vi "EF_EOG_Removal_PCA.vi"(8 "EOG":waveform(dbl)[](array[waveform]), 11 "EEG":waveform(dbl)[](array[waveform])) -> (3 "EEG out":waveform(dbl)[](array[waveform]))   [LabVIEW 2016, in "Feature Extraction.lvlib"]
uses:
  <vilib>/Analysis/baseanly.llb/Real A x B.vi
  <vilib>/addons/Time Series Analysis/Statistical Analysis.llb/TSA Principal Component Analysis (Waveform).vi
  Feature Extraction.lvlib
  <vilib>/Analysis/NI_AALBase.lvlib
  <vilib>/addons/_Advanced Signal Processing/NI_AdvSigProcTSA.lvlib
  4. Accuracy Assessment for EEG Classification/Classifier.lvlib
panel:
  out "Removed Principal Components":waveform(dbl)[](graph)
  out "Reconstructed EEG Signals":waveform(dbl)[](graph)
  out "Principal Components (PC)":waveform(dbl)[](graph)
  # "This VI is a part of BCI Design library, http://www.ru-bci.org \nCopyright © 2020, Sotnikov Peter, All rights reserved. License: GNU GPLv3"
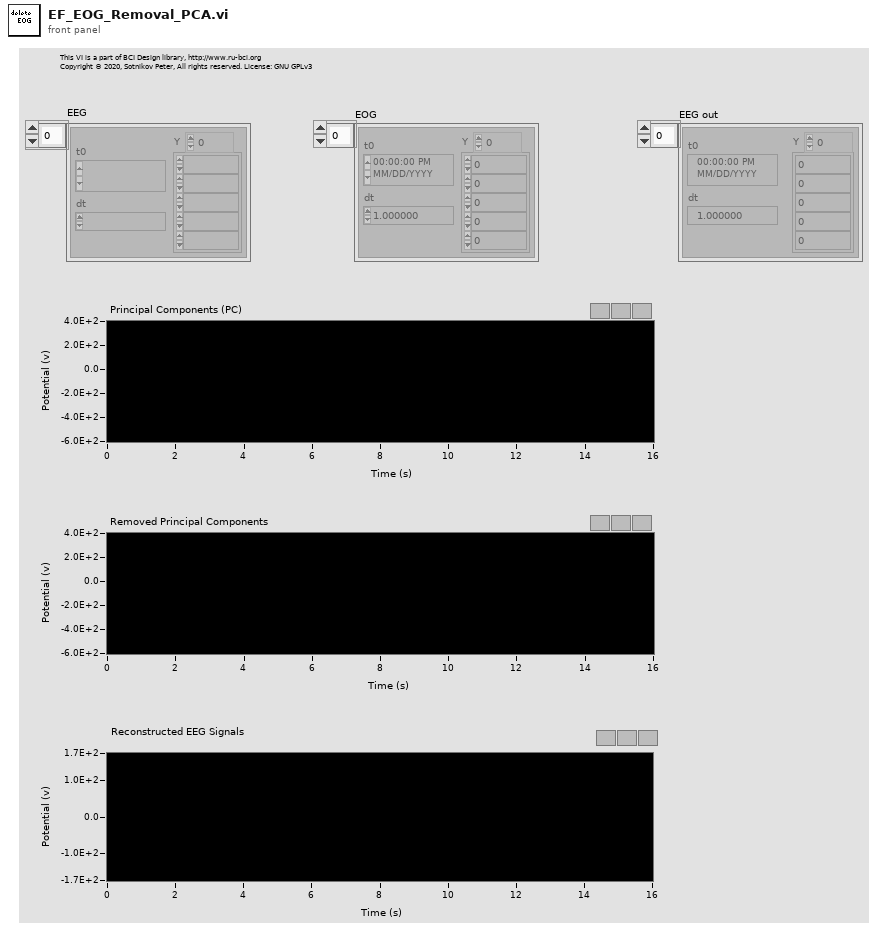
[diagram p1: front panel]
types:
  T1 = typedef "NI_Matrix.lvlib/RealMatrix.ctl" = dbl[][]
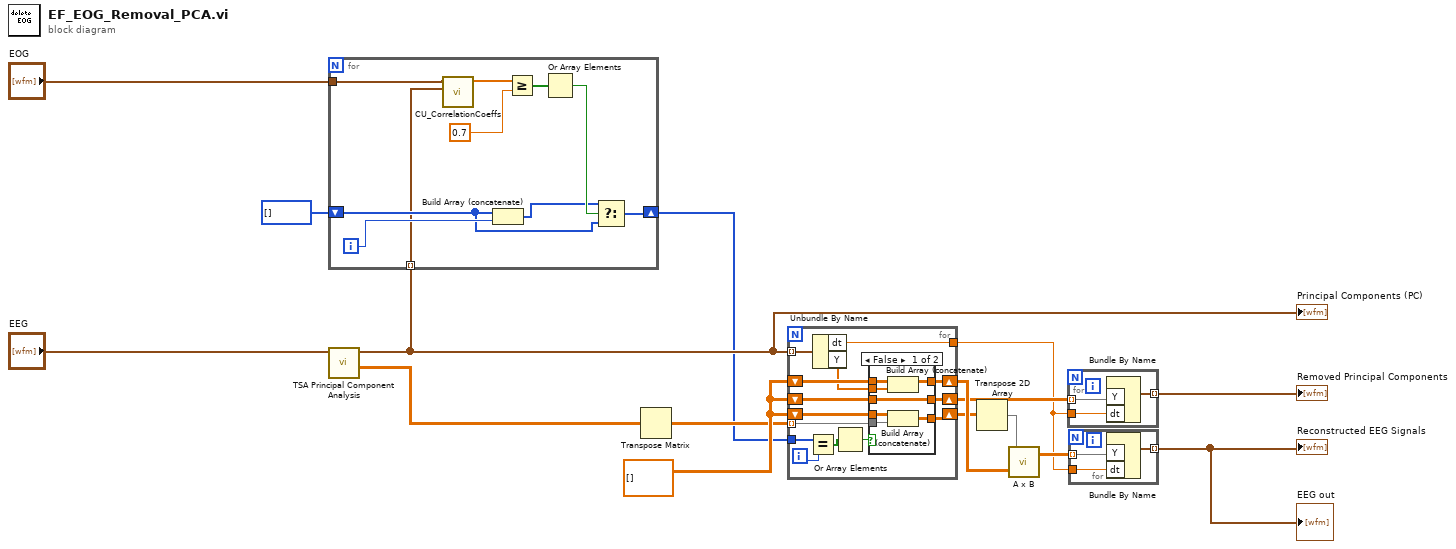
[diagram p0: block diagram]
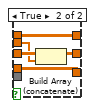
[diagram p2: hidden frame]
diagram:
  w15 = dbl[][] []
  n1 = call-poly <vilib>:"TSA Principal Component Analysis.vi"("Xt"="EEG") -> ("weights"=w5:dbl[][], "Xt out"=w8:waveform(dbl)[])  [unwired: 7 in, 2 out]
  "Principal Components (PC)" <- w8
  n2 = for {
    tunnel: "EOG" -> [w19]
    tunnel: w8 -> [w18] mode=indexing
    shift-right: [w20] -> w1
    shift-left: i32[] [] -> [w21]
    i -> [w23]
    n3 = call "CU_CorrelationCoeffs.vi"("Signal X"=w18, "Signal Y (Array)"=w19) -> ("CorrCoefficients"=w17:dbl[])  [unwired: 9 in]
    n4 = Build Array (concatenate)(w21, w23) -> (w22:i32[])
    n5 = Greater Or Equal?(x=w17, y=0.7) -> (x >= y?=w25:bool[])
    n6 = Or Array Elements(Boolean array=w25) -> (logical OR=w24:bool)
    n7 = Select(t=w22, s=w24, f=w21) -> (s? t:f=w20:i32[])
  }
  n8 = Transpose Matrix(1:w5) -> (0:w4:dbl[][])
  n9 = for {
    tunnel: w8 -> [w36] mode=indexing
    tunnel: w1 -> [w30]
    shift-right: [w37] -> w16
    shift-left: w15 -> [w38]
    shift-right: [w34] -> w13
    shift-left: w15 -> [w35]
    tunnel: w4 -> [w33] mode=indexing
    shift-right: [w31] -> w11
    shift-left: w15 -> [w32]
    tunnel: [w27] -> w9
    i -> [w29]
    n10 = Equal?(x=w30, y=w29) -> (x = y?=w40:bool[])
    n11 = Unbundle By Name(w36) -> ("dt"=w27:dbl, "Y"=w28:dbl[])
    n12 = Or Array Elements(Boolean array=w40) -> (logical OR=w39:bool)
    n13 = case shown="False" w39 {
      tunnel: w38 -> [w47 w52]
      tunnel: [w41 w52] -> w37
      tunnel: w28 -> [w46 w48]
      tunnel: w35 -> [w45 w51]
      tunnel: [w44 w51] -> w34
      tunnel: w33 -> [w43 _]
      tunnel: w32 -> [w42 w50]
      tunnel: [w42 w49] -> w31
      frame False {
        n14 = Build Array (concatenate)(w47, w46) -> (w41:dbl[][])
        n15 = Build Array (concatenate)(w45, w43) -> (w44:dbl[][])
      }
      frame True {
        n16 = Build Array (concatenate)(w50, w48) -> (w49:dbl[][])
      }
    }
  }
  n17 = Transpose 2D Array(2D array=w13) -> (transposed array=w14:dbl[][])
  n18 = call-poly <vilib>:"A x B.vi"("B"=w16, "A"=w14) -> ("A x B"=w12:T1)  [unwired: 1 out]
  n19 = for {
    tunnel: w11 -> [w55] mode=indexing
    tunnel: [w54] -> w10 mode=indexing
    tunnel: w9 -> [w53]
    n20 = Bundle By Name("Y"=w55, "dt"=w53) -> (w54:waveform(dbl))  [unwired: 1 out]
  }
  "Removed Principal Components" <- w10
  n21 = for {
    tunnel: w12 -> [w58] mode=indexing
    tunnel: [w57] -> w6 mode=indexing
    tunnel: w9 -> [w56]
    n22 = Bundle By Name("Y"=w58, "dt"=w56) -> (w57:waveform(dbl))  [unwired: 1 out]
  }
  "Reconstructed EEG Signals" <- w6
  "EEG out" <- w6
